vi "MGI Average (SGL[][]).vi"(0 "Single[][]":sgl[][](array[numeric]), 1 "Ignore NaN? (F)":bool) -> (2 "Average":sgl)   [LabVIEW 2016]
doc: "This VI computes and returns the average value of the given array of doubles.\n\nAuthored by Shawn D. Walpole\nsupport@mooregoodideas.com\nwww.mooregoodideas.com\n\nCopyright (c) 2010, Moore Good Ideas, Inc.\n\nAll rights reserved.\n\nRedistribution and use in source and binary forms, with or without modification, are permitted provided that the following conditions are met:\n\n * Redistributions of source code must retain the above copyright notice, this list of conditions and the following disclaimer.\n * Redistributions in binary form must reproduce the above copyright notice, this list of conditions and the following disclaimer in the documentation and/or other materials provided with the distribution.\n * Neither the name of Moore Good Ideas, Inc. nor the names of its contributors may be used to endorse or promote products derived from this software without specific prior written permission.\n\nTHIS SOFTWARE IS PROVIDED BY THE COPYRIGHT HOLDERS AND CONTRIBUTORS \"AS IS\" AND ANY EXPRESS OR IMPLIED WARRANTIES, INCLUDING, BUT NOT LIMITED TO, THE IMPLIED WARRANTIES OF MERCHANTABILITY AND FITNESS FOR A PARTICULAR PURPOSE ARE DISCLAIMED. IN NO EVENT SHALL THE COPYRIGHT OWNER OR CONTRIBUTORS BE LIABLE FOR ANY DIRECT, INDIRECT, INCIDENTAL, SPECIAL, EXEMPLARY, OR CONSEQUENTIAL DAMAGES (INCLUDING, BUT NOT LIMITED TO, PROCUREMENT OF SUBSTITUTE GOODS OR SERVICES; LOSS OF USE, DATA, OR PROFITS; OR BUSINESS INTERRUPTION) HOWEVER CAUSED AND ON ANY THEORY OF LIABILITY, WHETHER IN CONTRACT, STRICT LIABILITY, OR TORT (INCLUDING NEGLIGENCE OR OTHERWISE) ARISING IN ANY WAY OUT OF THE USE OF THIS SOFTWARE, EVEN IF ADVISED OF THE POSSIBILITY OF SUCH DAMAGE."
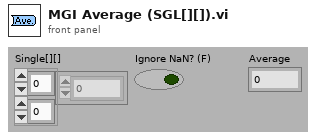
[diagram p1: front panel]
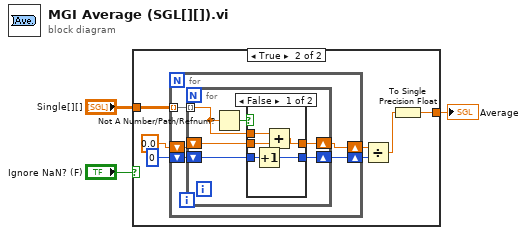
[diagram p0: block diagram]
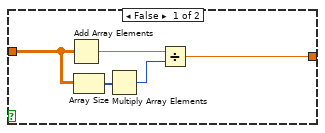
[diagram p2: hidden frame]
diagram:
  n1 = case shown="True" "Ignore NaN? (F)" {
    tunnel: "Single[][]" -> [w6 w13]
    tunnel: [w5 w9] -> w2
    frame False {
      n2 = Add Array Elements(numeric array=w6) -> (sum=w8:sgl)
      n3 = Array Size(array=w6) -> (size(s)=w7:i32[])
      n4 = Multiply Array Elements(1:w7) -> (0:w4:i32)
      n5 = Divide(x=w8, y=w4) -> (x/y=w5:sgl)
    }
    frame True {
      n6 = for {
        tunnel: w13 -> [w18] mode=indexing
        shift-right: [w16] -> w11
        shift-left: 0 -> [w20]
        shift-right: [w17] -> w12
        shift-left: 0.0 -> [w19]
        n7 = for {
          shift-right: [w21] -> w17
          shift-left: w19 -> [w23]
          shift-right: [w24] -> w16
          shift-left: w20 -> [w25]
          tunnel: w18 -> [w22] mode=indexing
          n8 = Not A Number/Path/Refnum?(number/path/refnum=w22) -> (NaN/Path/Refnum?=w26:bool)
          n9 = case shown="False" w26 {
            tunnel: w25 -> [w31 w32]
            tunnel: [w30 w32] -> w24
            tunnel: w23 -> [w29 w33]
            tunnel: w22 -> [w28 _]
            tunnel: [w27 w33] -> w21
            frame False {
              n10 = Increment(x=w31) -> (x+1=w30:i32)
              n11 = Add(x=w28, y=w29) -> (x+y=w27:dbl)
            }
            frame True {
            }
          }
        }
      }
      n12 = Divide(x=w12, y=w11) -> (x/y=w10:dbl)
      n13 = To Single Precision Float(number=w10) -> (single precision float=w9:sgl)
    }
  }
  "Average" <- w2
